vi "DAQmx Create Task.vi"(1 "new task name":string, 2 "auto cleanup":bool, 5 "task to copy":refnum<k21>, 7 "global virtual channels":refnum<k21>, 11 "error in":errorcluster) -> (4 "task out":refnum<k21>, 15 "error out":errorcluster)   [LabVIEW 2013]
doc: "Creates a task and adds virtual channels to that task if you specify them in the <B>global virtual channels</B> input. If you specify a <B>task to copy</B>, this VI duplicates the configuration of the specified task in the newly created task before it adds any additional global virtual channels."
uses:
  nilvaiu.dll
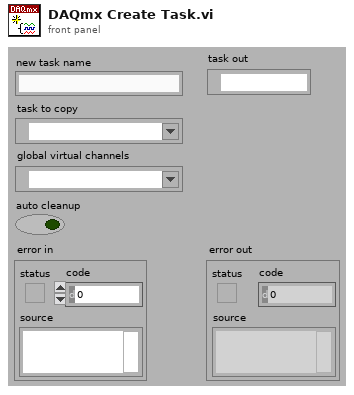
[diagram p1: front panel]
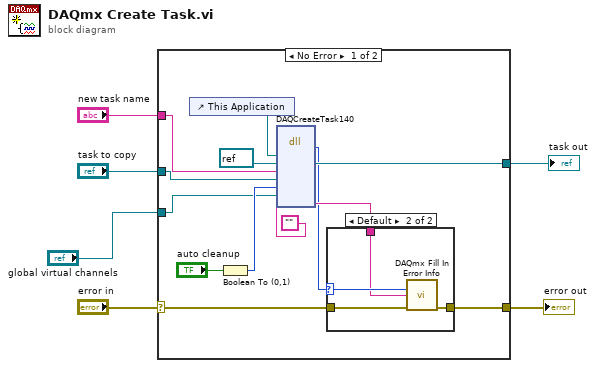
[diagram p0: block diagram]
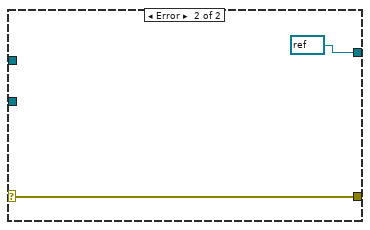
[diagram p3: hidden frame]
diagram:
  n1 = case shown="No Error" "error in" {
    selector: "error in" -> [w19 w26]
    tunnel: [w17 w26] -> w4
    tunnel: "new task name" -> [w15 _]
    tunnel: "task to copy" -> [w14 _]
    tunnel: "global virtual channels" -> [w12 _]
    tunnel: [w9 refnum<k21> refnum] -> w1
    frame No Error {
      n2 = control-ref of="This Application"() -> (w7:refnum<vi>)
      n3 = Boolean To (0,1)(Boolean="auto cleanup") -> (0, 1=w13:i16)
      n4 = dll-call lib="nilvaiu.*" fn="DAQCreateTask140"("lvAppReference"=w7, "taskRefObjectPtr"=refnum<k21> refnum, "newTaskName"=w15, "taskToCopy"=w14, "autoCleanup"=w13, "channels"=w12, "extendedErrorInfo"="") -> (w8:i32, "taskRefObjectPtr"=w9:refnum<k21>, "extendedErrorInfo"=w10:string)  [unwired: 5 in, 5 out]
      n5 = case shown="Default" w8 {
        selector: w8 -> [_ w22]
        tunnel: w19 -> [w20 w24]
        tunnel: [w20 w23] -> w17
        tunnel: w10 -> [_ w21]
        frame 0 {
        }
        frame Default {
          n6 = call "DAQmx Fill In Error Info.vi"("status code"=w22, "extended error info"=w21, "error in"=w24) -> ("error out"=w23:errorcluster)  [unwired: 1 in, 11 out]
        }
      }
    }
    frame Error {
    }
  }
  "error out" <- w4
  "task out" <- w1
